vi "Main.vi"() -> ()   [LabVIEW 2026]
uses:
  Controls/Hall_Calls.ctl
  Controls/Car_Calls.ctl
  Controls/Elevator_Fleet.ctl
  Controls/Elevator_Status.ctl
  Controls/Door_Status_Enum.ctl
  Controls/Occupy_Status.ctl
  Controls/Floor_Status.ctl
  Controls/Motion_Status_Enum.ctl
  Controls/Car_Calls_Status.ctl
  Controls/Hall_Calls_Status.ctl
  Support VIs/Message Queue/Enqueue Message (Single).vi
  <vilib>/Utility/error.llb/Error Cluster From Error Code.vi
  <vilib>/ErrorRing/Error Ring.xnode
  Support VIs/Message Queue/Message Queue.lvlib
  Support VIs/User Event - Stop/User Event - Stop.lvlib
panel:
  out "Elevator Fleet":T1
  out "data":string
  in  "Exit":bool
  in  "Car Calls":T9
  in  "Hall Calls Up/Down":T10
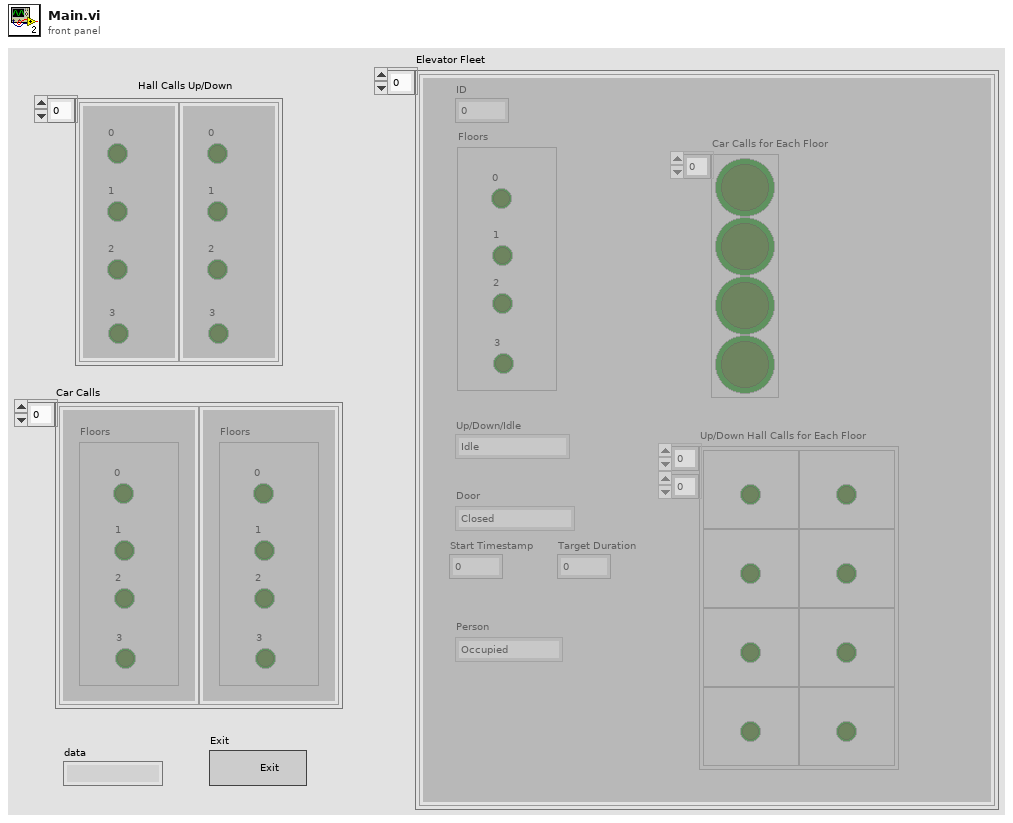
[diagram p1: front panel]
types:
  T1 = typedef "Elevator_Fleet.ctl" = T2[]
  T2 = typedef "Elevator_Status.ctl" = cluster{"Door":T3, "Person":T4, "Floors":T5, "Up/Down/Idle":T6, "Car Calls for Each Floor":T7, "Up/Down Hall Calls for Each Floor":T8, "ID":i32, "Start Timestamp":u32, "Target Duration":dbl}
  T3 = typedef "Door_Status_Enum.ctl" = enum16{"Closed", "Open", "Opening", "Closing"}
  T4 = typedef "Occupy_Status.ctl" = enum16{"Occupied", "Empty"}
  T5 = typedef "Floor_Status.ctl" = cluster{"0":bool, "1":bool, "2":bool, "3":bool}
  T6 = typedef "Motion_Status_Enum.ctl" = enum16{"Idle", "Up", "Down"}
  T7 = typedef "Car_Calls_Status.ctl" = bool[]
  T8 = typedef "Hall_Calls_Status.ctl" = cluster{bool}[][]
  T9 = typedef "Car_Calls.ctl" = cluster{"Floors":cluster{"0":bool, "1":bool, "2":bool, "3":bool}}[]
  T10 = typedef "Hall_Calls.ctl" = cluster{"0":bool, "1":bool, "2":bool, "3":bool}[]
  T11 = typedef "Message Queue.lvlib/All Message Queues.ctl" = cluster{"UI":refnum<queue>, "Acquisition":refnum<queue>, "Logging":refnum<queue>}
  T12 = enum16{"Check for Any Floor - Car Call", "Check for Specific Floor - Car Call", "Check for Any Floor - Hall Call", "Check for Specific Floor - Hall Call"}
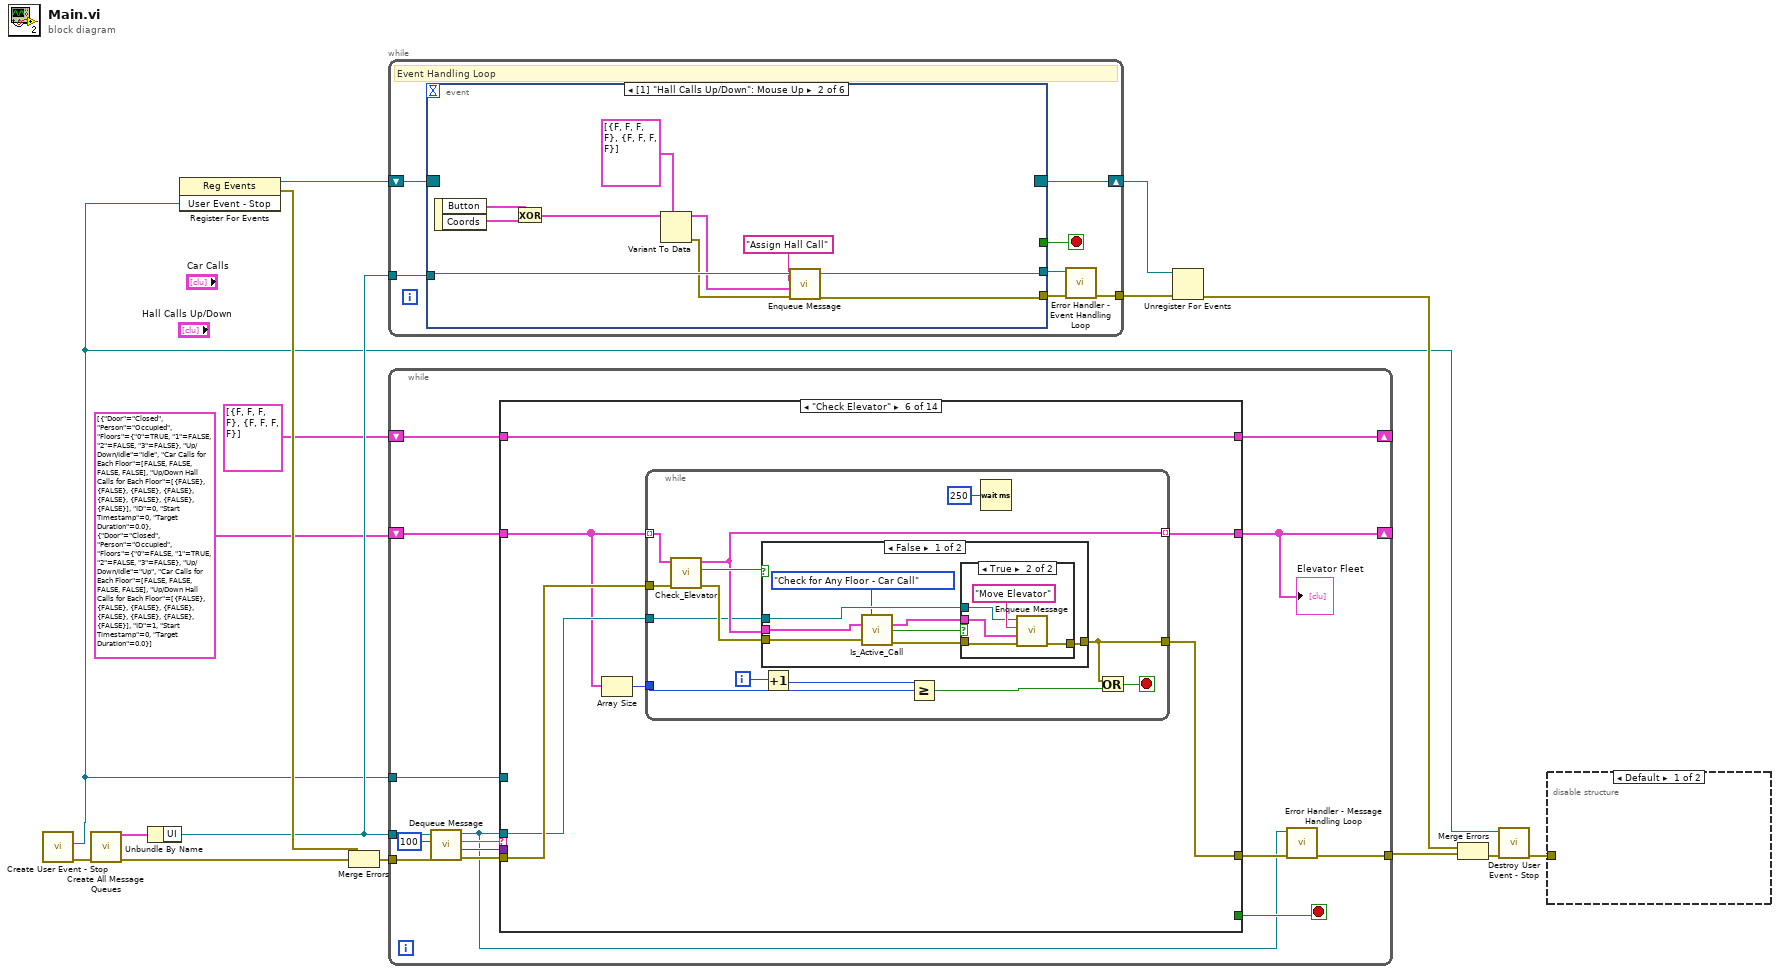
[diagram p0: block diagram]
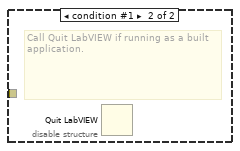
[diagram p2: hidden frame]
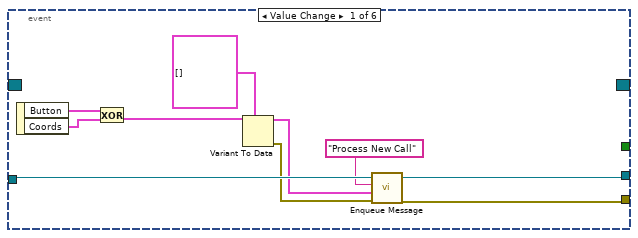
[diagram p3: hidden frame]
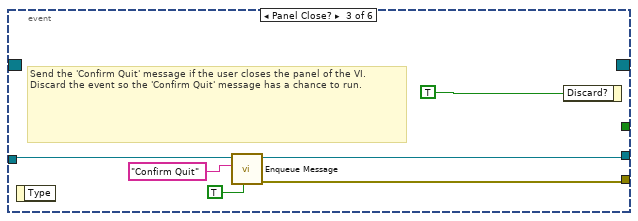
[diagram p4: hidden frame]
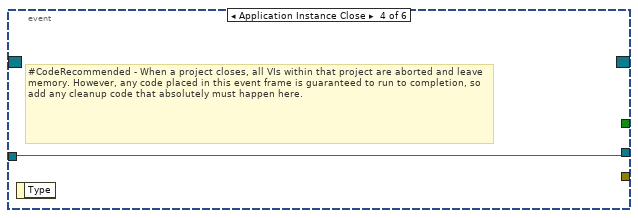
[diagram p5: hidden frame]
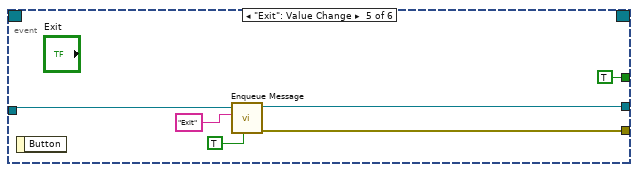
[diagram p6: hidden frame]
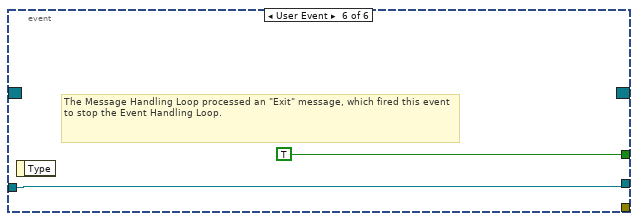
[diagram p7: hidden frame]
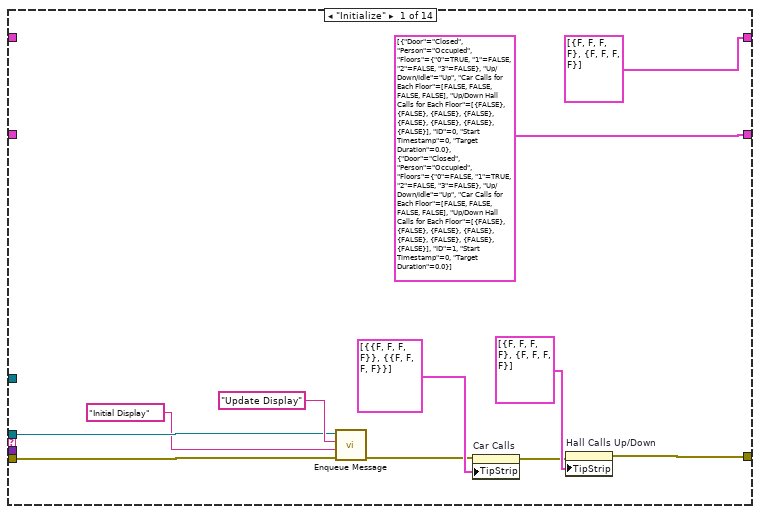
[diagram p8: hidden frame]
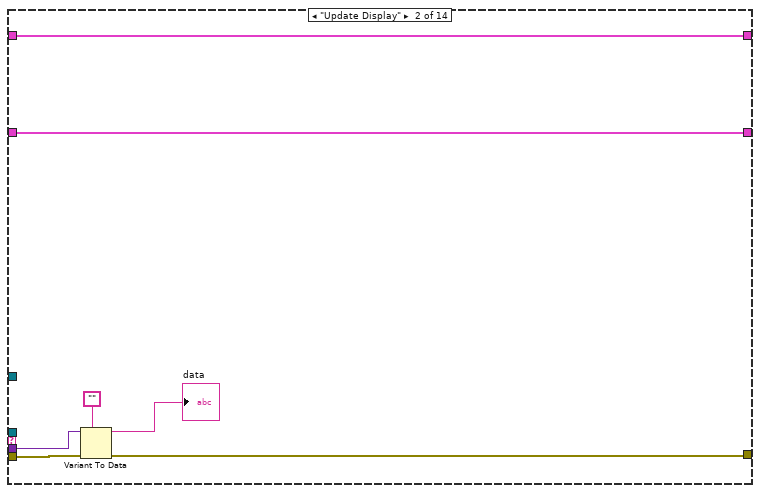
[diagram p9: hidden frame]
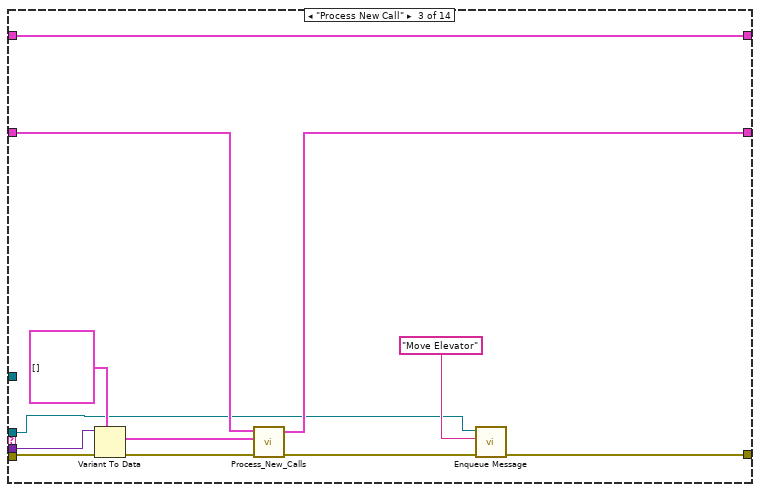
[diagram p10: hidden frame]
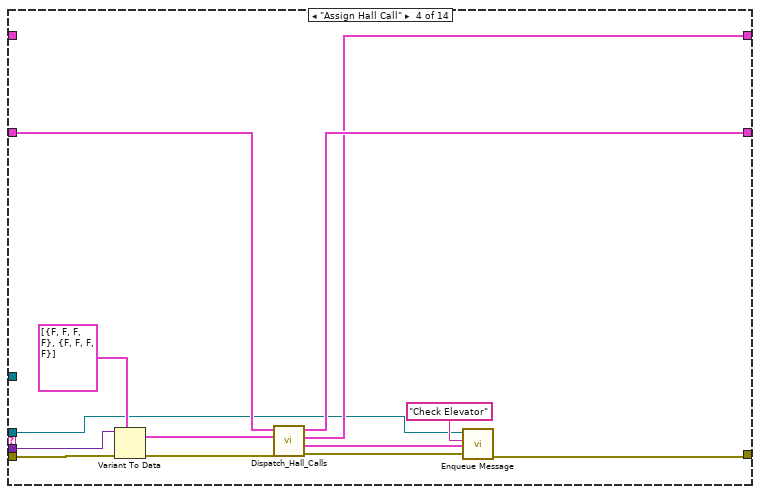
[diagram p11: hidden frame]
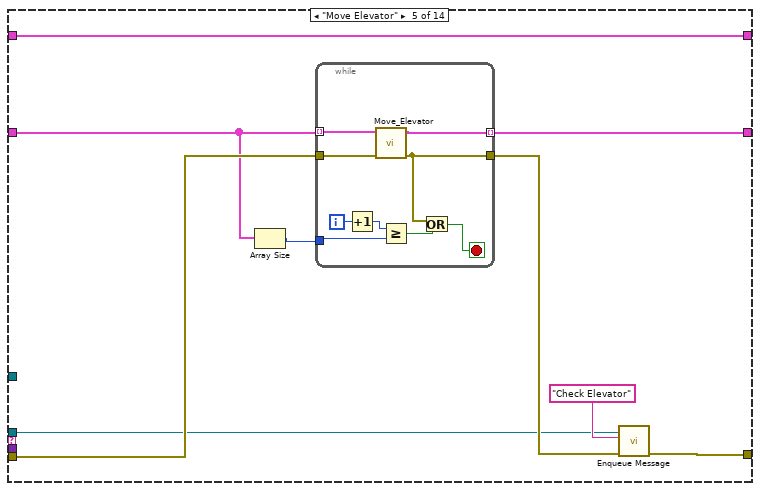
[diagram p12: hidden frame]
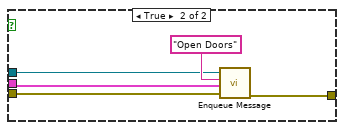
[diagram p14: hidden frame]
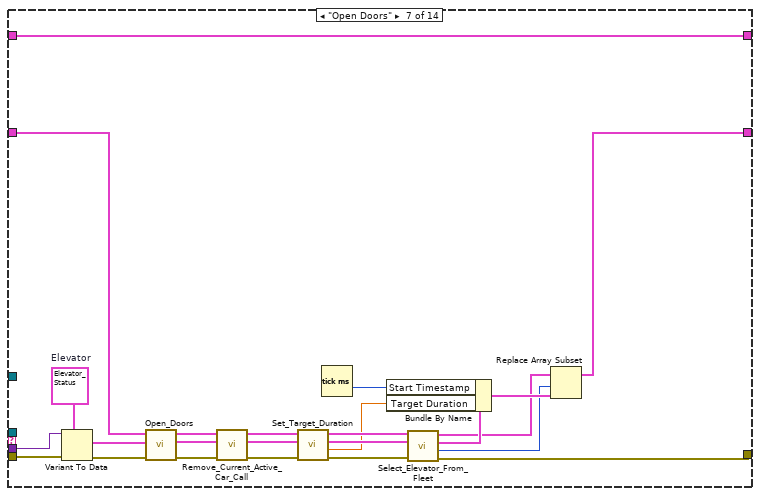
[diagram p15: hidden frame]
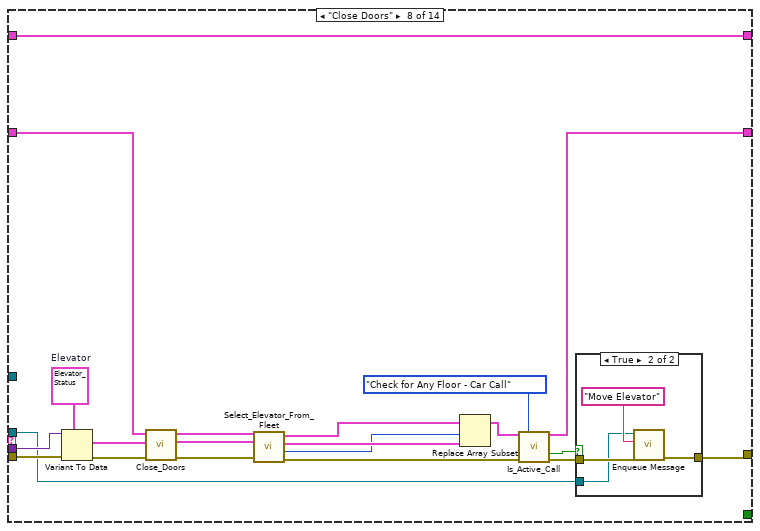
[diagram p16: hidden frame]
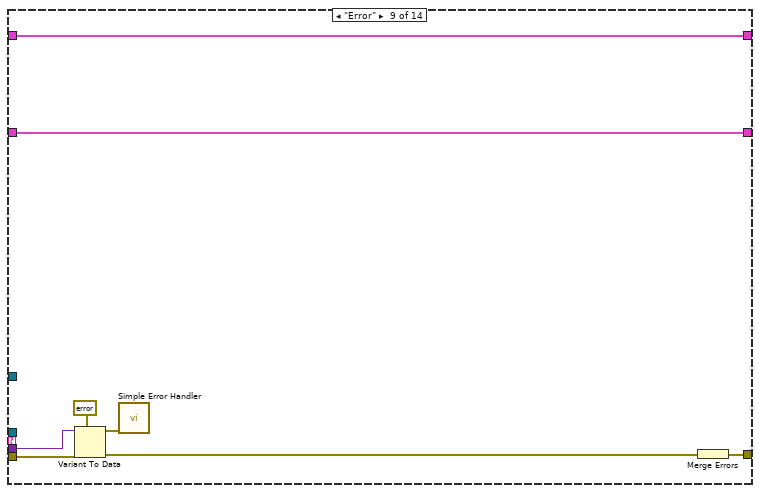
[diagram p18: hidden frame]
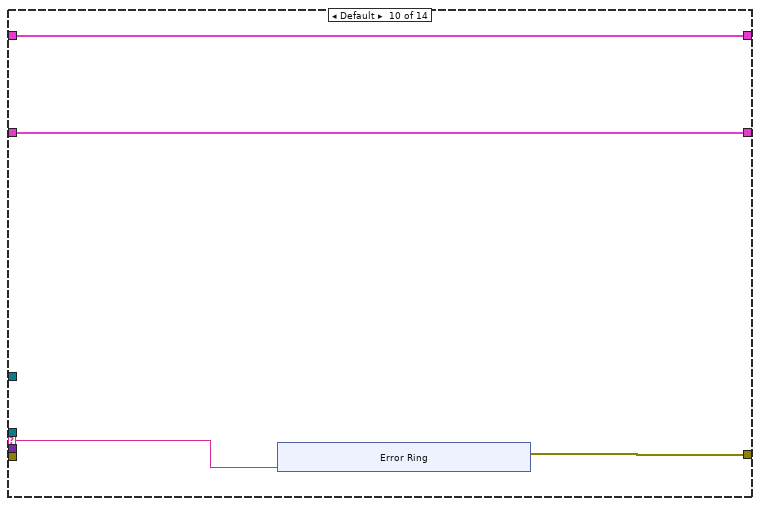
[diagram p19: hidden frame]
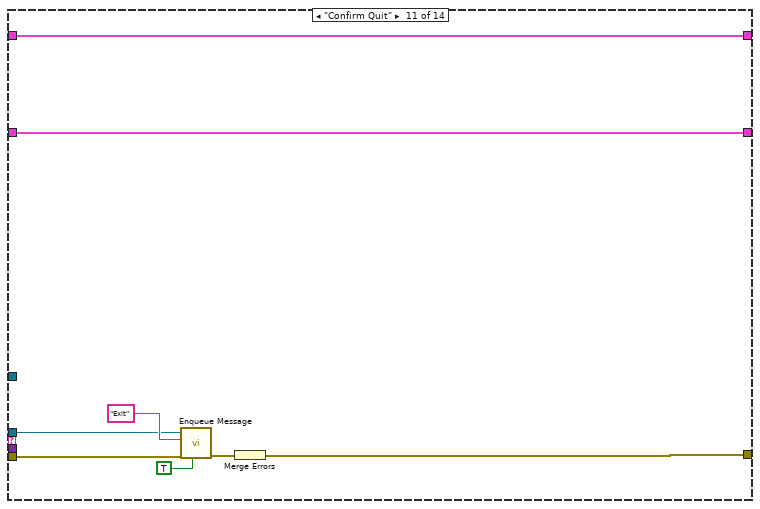
[diagram p20: hidden frame]
diagram:
  n1 = call "Create User Event - Stop.vi"() -> ("error out"=w16:errorcluster, "User Event - Stop"=w3:refnum<user-event>)  [unwired: 9 in, 1 out]
  n2 = call "Create All Message Queues.vi"("error in (no error)"=w16) -> ("error out"=w14:errorcluster, "Message Queues out"=w15:T11)  [unwired: 9 in]
  n3 = Unbundle By Name(w15) -> ("UI"=w10:refnum<queue>)
  n4 = register-events(w3) -> (reference out=w13:refnum<event-registration>, error out=w12:errorcluster)  [unwired: 2 in]
  n5 = Merge Errors(w12, w14) -> (w11:errorcluster)
  n6 = while {
    shift-right: [w23] -> w6
    shift-left: w13 -> [w18]
    tunnel: [w19] -> w7
    tunnel: w10 -> [w17]
    stop <- w21 stop-if-true
    # "Event Handling Loop"
    n7 = event shown="[1] \"Hall Calls Up/Down\": Mouse Up" {
      selector: w18 -> [_ _ _ _ _ _]
      dyn-events: [_ _ _ _ _ _] -> w23
      timeout: _ -> [_ _ _ _ _ _]
      tunnel: [_ _ _ _ TRUE ("Discard?") TRUE ("Discard?")] -> w21
      tunnel: [w32 w42 w48 _ w56 _] -> w22
      tunnel: [w33 w43 w47 w50 w55 w57] -> w20
      tunnel: w17 -> [w31 w41 w44 w50 w52 w57]
      event Value Change {
        n8 = event-data() -> ("Button"=w26:T9, "Coords"=w25:T9)  [unwired: 1 in]
        n9 = Exclusive Or(1:w25, 2:w26) -> (0:w24:T9)
        n10 = Variant To Data(type=T9 [] ("x .xor. y?"), Variant=w24) -> (data=w29:T9, error out=w28:errorcluster)  [unwired: 1 in]
        n11 = call-poly "Enqueue Message.vi"("error in (no error)"=w28, "Message Data"=w29, "Message"="Process New Call", "Message Queue"=w31) -> ("error out"=w32:errorcluster, "dup Message Queue"=w33:refnum<queue>)  [unwired: 6 in]
      }
      event Value Change {
        n12 = event-data() -> ("Button"=w37:T10, "Coords"=w36:T10)  [unwired: 1 in]
        n13 = Exclusive Or(1:w36, 2:w37) -> (0:w35:T10)
        n14 = Variant To Data(type=T10 [{"0"=FALSE, "1"=FALSE, "2"=FALSE, "3"=FALSE}, {"0"=FALSE, "1"=FALSE, "2"=FALSE, "3"=FALSE}] ("x .xor. y?"), Variant=w35) -> (data=w39:T10, error out=w38:errorcluster)  [unwired: 1 in]
        n15 = call-poly "Enqueue Message.vi"("error in (no error)"=w38, "Message Data"=w39, "Message"="Assign Hall Call", "Message Queue"=w41) -> ("error out"=w42:errorcluster, "dup Message Queue"=w43:refnum<queue>)  [unwired: 6 in]
      }
      event Panel Close? {
        # "Send the 'Confirm Quit' message if the user closes the panel of the VI. Discard the event so the 'Confirm Quit' message has a chance to run."
        n16 = event-data() -> ()  [unwired: 1 in, 1 out]
        n17 = call-poly "Enqueue Message.vi"("Priority Message? (F)"=TRUE, "Message"="Confirm Quit", "Message Queue"=w44) -> ("error out"=w48:errorcluster, "dup Message Queue"=w47:refnum<queue>)  [unwired: 7 in]
        n18 = event-data("Discard?"=TRUE) -> ()  [unwired: 1 in, 1 out]
      }
      event Application Instance Close {
        # "#CodeRecommended - When a project closes, all VIs within that project are aborted and leave memory. However, any code placed in this event frame is guaranteed to run to completion, so add any cleanup code that absolutely must happen here."
        n19 = event-data() -> ()  [unwired: 1 in, 1 out]
      }
      event "Exit": Value Change {
        n20 = event-data() -> ()  [unwired: 1 in, 1 out]
        n21 = call-poly "Enqueue Message.vi"("Priority Message? (F)"=TRUE, "Message"="Exit", "Message Queue"=w52) -> ("error out"=w56:errorcluster, "dup Message Queue"=w55:refnum<queue>)  [unwired: 7 in]
      }
      event User Event {
        # "The Message Handling Loop processed an \"Exit\" message, which fired this event to stop the Event Handling Loop."
        n22 = event-data() -> ()  [unwired: 1 in, 1 out]
      }
    }
    n23 = call "Error Handler - Event Handling Loop.vi"("error in (no error)"=w22, "Message Queue"=w20) -> ("dup error in"=w19:errorcluster)  [unwired: 8 in, 1 out]
  }
  n24 = while {
    tunnel: w10 -> [w72]
    tunnel: w11 -> [w71]
    tunnel: w3 -> [w67]
    tunnel: [w65] -> w8
    shift-right: [w63] -> _
    shift-left: T1 [{"Door"=enum."Closed", "Person"=enum."Occupied", "Floors"={"0"=TRUE, "1"=FALSE, "2"=FALSE, "3"=FALSE}, "Up/Down/Idle"=enum."Idle", "Car Calls for Each Floor"=[FALSE, FALSE, FALSE, FALSE], "Up/Down Hall Calls for Each Floor"=[[{FALSE}, {FALSE}], [{FALSE}, {FALSE}], [{FALSE}, {FALSE}], [{FALSE}, {FALSE}]], "ID"=0, "Start Timestamp"=0, "Target Duration"=0.0}, {"Door"=enum."Closed", "Person"=enum."Occupied", "Floors"={"0"=FALSE, "1"=TRUE, "2"=FALSE, "3"=FALSE}, "Up/Down/Idle"=enum."Up", "Car Calls for Each Floor"=[FALSE, FALSE, FALSE, FALSE], "Up/Down Hall Calls for Each Floor"=[[{FALSE}, {FALSE}], [{FALSE}, {FALSE}], [{FALSE}, {FALSE}], [{FALSE}, {FALSE}]], "ID"=1, "Start Timestamp"=0, "Target Duration"=0.0}] ("Elevator Fleet") -> [w73]
    shift-right: [w61] -> _
    shift-left: T10 [{"0"=FALSE, "1"=FALSE, "2"=FALSE, "3"=FALSE}, {"0"=FALSE, "1"=FALSE, "2"=FALSE, "3"=FALSE}] ("x .xor. y?") -> [w62]
    stop <- w64 stop-if-true
    n25 = call "Dequeue Message.vi"("error in (no error)"=w71, "Timeout (ms)"=100, "Message Queue"=w72) -> ("error out"=w69:errorcluster, "Message Data"=w68:variant, "Message"=w70:string, "dup Message Queue"=w60:refnum<queue>)  [unwired: 5 in]
    n26 = case shown="\"Check Elevator\"" w70 {
      selector: w70 -> [_ _ _ _ _ _ _ _ _ w235 _ _ _ _]
      tunnel: w73 -> [_ w86 w98 w113 w118 w136 w193 w214 w225 w233 w244 w252 w257 w300]
      tunnel: w60 -> [w82 _ w92 w105 w119 w137 _ w199 _ _ w245 _ w260 w302]
      tunnel: w69 -> [w83 w90 w100 w116 w121 w140 w196 w217 w229 _ w246 w254 w259 w298]
      tunnel: w68 -> [_ w89 w102 w115 _ _ w195 w216 w228 _ _ _ _ w301]
      tunnel: [w74 w88 w95 w108 w122 w138 w185 w201 w226 w234 w247 w253 w258 w305] -> w66
      tunnel: w67 -> [_ _ _ _ _ _ _ _ _ _ _ _ _ w303]
      tunnel: [_ _ _ _ _ _ _ _ _ _ _ _ _ TRUE] -> w64
      tunnel: [T1 [{"Door"=enum."Closed", "Person"=enum."Occupied", "Floors"={"0"=TRUE, "1"=FALSE, "2"=FALSE, "3"=FALSE}, "Up/Down/Idle"=enum."Up", "Car Calls for Each Floor"=[FALSE, FALSE, FALSE, FALSE], "Up/Down Hall Calls for Each Floor"=[[{FALSE}, {FALSE}], [{FALSE}, {FALSE}], [{FALSE}, {FALSE}], [{FALSE}, {FALSE}]], "ID"=0, "Start Timestamp"=0, "Target Duration"=0.0}, {"Door"=enum."Closed", "Person"=enum."Occupied", "Floors"={"0"=FALSE, "1"=TRUE, "2"=FALSE, "3"=FALSE}, "Up/Down/Idle"=enum."Up", "Car Calls for Each Floor"=[FALSE, FALSE, FALSE, FALSE], "Up/Down Hall Calls for Each Floor"=[[{FALSE}, {FALSE}], [{FALSE}, {FALSE}], [{FALSE}, {FALSE}], [{FALSE}, {FALSE}]], "ID"=1, "Start Timestamp"=0, "Target Duration"=0.0}] ("Elevator Fleet") w86 w97 w114 w124 w139 w187 w200 w225 w233 w244 w252 w255 w300] -> w63
      tunnel: w62 -> [_ w85 w103 _ w125 w141 w197 w218 w224 w232 w243 w251 w261 w299]
      tunnel: [T10 [{"0"=FALSE, "1"=FALSE, "2"=FALSE, "3"=FALSE}, {"0"=FALSE, "1"=FALSE, "2"=FALSE, "3"=FALSE}] ("x .xor. y?") w85 w103 w110 w125 w141 w197 w218 w224 w232 w243 w251 w261 w299] -> w61
      frame "Initialize" {
        n27 = call-poly "Enqueue Message.vi"("error in (no error)"=w83, "Message Data"="Initial Display" ("Message"), "Message"="Update Display", "Message Queue"=w82) -> ("error out"=w77:errorcluster)  [unwired: 6 in, 1 out]
        n28 = property on="Car Calls" class="Arr (strict)"(error in=w77, "TipStrip"=T9 [{"Floors"={"0"=FALSE, "1"=FALSE, "2"=FALSE, "3"=FALSE}}, {"Floors"={"0"=FALSE, "1"=FALSE, "2"=FALSE, "3"=FALSE}}] ("Car Calls")) -> (error out=w75:errorcluster)  [unwired: 1 in, 1 out]
        n29 = property on="Hall Calls Up/Down" class="Arr (strict)"(error in=w75, "TipStrip"=T10 [{"0"=FALSE, "1"=FALSE, "2"=FALSE, "3"=FALSE}, {"0"=FALSE, "1"=FALSE, "2"=FALSE, "3"=FALSE}] ("Hall Calls Up/Down")) -> (error out=w74:errorcluster)  [unwired: 1 in, 1 out]
      }
      frame "Update Display" {
        n30 = Variant To Data(error in=w90, type="", Variant=w89) -> (data=→"data":string, error out=w88:errorcluster)
      }
      frame "Process New Call" {
        n31 = Variant To Data(error in=w100, type=T9 [] ("x .xor. y?"), Variant=w102) -> (data=w99:T9, error out=w94:errorcluster)
        n32 = call "Process_New_Calls.vi"("error in (no error)"=w94, "Car Calls in"=w99, "Elevator Fleet in"=w98) -> ("error out"=w93:errorcluster, "Elevator Fleet out"=w97:T1)  [unwired: 7 in]
        n33 = call-poly "Enqueue Message.vi"("error in (no error)"=w93, "Message"="Move Elevator", "Message Queue"=w92) -> ("error out"=w95:errorcluster)  [unwired: 7 in, 1 out]
      }
      frame "Assign Hall Call" {
        n34 = Variant To Data(error in=w116, type=T10 [{"0"=FALSE, "1"=FALSE, "2"=FALSE, "3"=FALSE}, {"0"=FALSE, "1"=FALSE, "2"=FALSE, "3"=FALSE}] ("x .xor. y?"), Variant=w115) -> (data=w111:T10, error out=w107:errorcluster)
        n35 = call "Dispatch_Hall_Calls.vi"("error in (no error)"=w107, "Hall Calls Up/Down In"=w111, "Elevator Fleet in"=w113) -> ("error out"=w106:errorcluster, "Elevator Called"=w104:T2, "Hall Calls Up/Down Out"=w110:T10, "Elevator Fleet out"=w114:T1)  [unwired: 5 in]
        n36 = call-poly "Enqueue Message.vi"("error in (no error)"=w106, "Message Data"=w104, "Message"="Check Elevator", "Message Queue"=w105) -> ("error out"=w108:errorcluster)  [unwired: 6 in, 1 out]
      }
      frame "Move Elevator" {
        n37 = Array Size(array=w118) -> (size(s)=w117:i32)
        n38 = while {
          tunnel: w118 -> [w134] mode=indexing
          tunnel: [w133] -> w124 mode=indexing
          tunnel: w121 -> [w132]
          tunnel: [w129] -> w120
          tunnel: w117 -> [w131]
          i -> [w127]
          stop <- w130 stop-if-true
          n39 = Increment(x=w127) -> (x+1=w126:i32)
          n40 = call "Move_Elevator.vi"("error in (no error)"=w132, "Elevator in"=w134) -> ("error out"=w129:errorcluster, "Elevator out"=w133:T2)  [unwired: 8 in]
          n41 = Greater Or Equal?(x=w126, y=w131) -> (x >= y?=w128:bool)
          n42 = Or(x=w129, y=w128) -> (x .or. y?=w130:bool)
        }
        n43 = call-poly "Enqueue Message.vi"("error in (no error)"=w120, "Message"="Check Elevator", "Message Queue"=w119) -> ("error out"=w122:errorcluster)  [unwired: 7 in, 1 out]
      }
      frame "Check Elevator" {
        n44 = Array Size(array=w136) -> (size(s)=w135:i32)
        n45 = while {
          tunnel: w140 -> [w154]
          tunnel: [w151] -> w139 mode=indexing
          tunnel: [w147] -> w138
          tunnel: w137 -> [w150]
          tunnel: w136 -> [w149] mode=indexing
          tunnel: w135 -> [w148]
          i -> [w143]
          stop <- w145 stop-if-true
          n46 = call "Check_Elevator.vi"("error in (no error)"=w154, "Elevator in"=w149) -> ("error out"=w152:errorcluster, "Open Doors?"=w153:bool, "Elevator out"=w151:T2)  [unwired: 7 in]
          n47 = case shown="False" w153 {
            tunnel: w152 -> [w161 w172]
            tunnel: [w157 w171] -> w147
            tunnel: w151 -> [w159 w170]
            tunnel: w150 -> [w162 w169]
            frame False {
              n48 = call "Is_Active_Call.vi"("Enum"=T12."Check for Any Floor - Car Call", "Elevator in"=w159, "error in (no error)"=w161) -> ("Elevator out"=w156:T2, "Active Call?"=w158:bool, "error out"=w160:errorcluster)  [unwired: 8 in, 2 out]
              n49 = case shown="True" w158 {
                tunnel: w162 -> [_ w167]
                tunnel: w160 -> [w163 w166]
                tunnel: [w163 w165] -> w157
                tunnel: w156 -> [_ w164]
                frame False {
                }
                frame True {
                  n50 = call-poly "Enqueue Message.vi"("error in (no error)"=w166, "Message Data"=w164, "Message"="Move Elevator", "Message Queue"=w167) -> ("error out"=w165:errorcluster)  [unwired: 6 in, 1 out]
                }
              }
            }
            frame True {
              n51 = call-poly "Enqueue Message.vi"("error in (no error)"=w172, "Message Data"=w170, "Message"="Open Doors", "Message Queue"=w169) -> ("error out"=w171:errorcluster)  [unwired: 6 in, 1 out]
            }
          }
          n52 = Increment(x=w143) -> (x+1=w142:i32)
          n53 = Greater Or Equal?(x=w142, y=w148) -> (x >= y?=w146:bool)
          n54 = Wait (ms)(milliseconds to wait=u32 250) -> ()  [unwired: 1 out]
          n55 = Or(x=w147, y=w146) -> (x .or. y?=w145:bool)
        }
      }
      frame "Open Doors" {
        w194 = T2 {"Door"=enum."Closed", "Person"=enum."Occupied", "Floors"={"0"=FALSE, "1"=FALSE, "2"=FALSE, "3"=FALSE}, "Up/Down/Idle"=enum."Idle", "Car Calls for Each Floor"=[], "Up/Down Hall Calls for Each Floor"=[], "ID"=0, "Start Timestamp"=0, "Target Duration"=0.0}  # Elevator
        n56 = Variant To Data(error in=w196, type=w194, Variant=w195) -> (data=w192:T2, error out=w191:errorcluster)
        n57 = call "Open_Doors.vi"("error in (no error)"=w191, "Elevator in"=w192, "Elevator Fleet in"=w193) -> ("error out"=w175:errorcluster, "Elevator out"=w177:T2, "Elevator Fleet out"=w179:T1)  [unwired: 6 in]
        n58 = call "Remove_Current_Active_Car_Call.vi"("error in (no error)"=w175, "Elevator in"=w177, "Elevator Fleet in"=w179) -> ("error out"=w174:errorcluster, "Elevator out"=w176:T2, "Elevator Fleet out"=w178:T1)  [unwired: 6 in]
        n59 = call "Set_Target_Duration.vi"("error in (no error)"=w174, "Elevator in"=w176, "Elevator Fleet in"=w178) -> ("error out"=w186:errorcluster, "Target Duration"=w181:dbl, "Elevator out"=w182:T2, "Elevator Fleet out"=w183:T1)  [unwired: 5 in]
        n60 = Tick Count (ms)() -> (millisecond timer value=w189:u32)
        n61 = call "Select_Elevator_From_Fleet.vi"("error in (no error)"=w186, "Elevator in"=w182, "Elevator Fleet in"=w183) -> ("error out"=w185:errorcluster, "ID"=w184:i32, "Elevator out"=w190:T2, "Elevator Fleet out"=w180:T1)  [unwired: 5 in]
        n62 = Bundle By Name(cluster=w190, "Start Timestamp"=w189, "Target Duration"=w181) -> (w188:T2)
        n63 = Replace Array Subset(array=w180, new element=w188, index=w184) -> (w187:T1)
      }
      frame "Close Doors" {
        w215 = T2 {"Door"=enum."Closed", "Person"=enum."Occupied", "Floors"={"0"=FALSE, "1"=FALSE, "2"=FALSE, "3"=FALSE}, "Up/Down/Idle"=enum."Idle", "Car Calls for Each Floor"=[], "Up/Down Hall Calls for Each Floor"=[], "ID"=0, "Start Timestamp"=0, "Target Duration"=0.0}  # Elevator
        n64 = Variant To Data(error in=w217, type=w215, Variant=w216) -> (data=w213:T2, error out=w212:errorcluster)
        n65 = call "Close_Doors.vi"("error in (no error)"=w212, "Elevator in"=w213, "Elevator Fleet in"=w214) -> ("error out"=w209:errorcluster, "Elevator out"=w210:T2, "Elevator Fleet out"=w211:T1)  [unwired: 6 in]
        n66 = call "Select_Elevator_From_Fleet.vi"("error in (no error)"=w209, "Elevator in"=w210, "Elevator Fleet in"=w211) -> ("error out"=w205:errorcluster, "ID"=w206:i32, "Elevator out"=w207:T2, "Elevator Fleet out"=w208:T1)  [unwired: 5 in]
        n67 = Replace Array Subset(array=w208, new element=w207, index=w206) -> (w204:T1)
        n68 = call "Is_Active_Call.vi"("Elevator Fleet in"=w204, "Enum"=T12."Check for Any Floor - Car Call", "error in (no error)"=w205) -> ("Elevator Fleet out"=w200:T1, "Active Call?"=w203:bool, "error out"=w202:errorcluster)  [unwired: 8 in, 2 out]
        n69 = case shown="True" w203 {
          tunnel: w202 -> [w219 w222]
          tunnel: [w219 w221] -> w201
          tunnel: w199 -> [_ w220]
          frame False {
          }
          frame True {
            n70 = call-poly "Enqueue Message.vi"("error in (no error)"=w222, "Message"="Move Elevator", "Message Queue"=w220) -> ("error out"=w221:errorcluster)  [unwired: 7 in, 1 out]
          }
        }
      }
      frame "Error" {
        n71 = Variant To Data(error in=w229, type=errorcluster {"status"=FALSE, "code"=0, "source"=""} ("error constant"), Variant=w228) -> (data=w231:errorcluster, error out=w227:errorcluster)
        n72 = call <vilib>:"Simple Error Handler.vi"("error in (no error)"=w231) -> ()  [unwired: 4 in, 5 out]
        n73 = Merge Errors(w227) -> (w226:errorcluster)
      }
      frame Default {
        n74 = xnode "Error Ring"("parameter 0"=w235) -> ("error out"=w234:errorcluster)
      }
      frame "Confirm Quit" {
        n75 = call-poly "Enqueue Message.vi"("Priority Message? (F)"=TRUE, "error in (no error)"=w246, "Message"="Exit", "Message Queue"=w245) -> ("error out"=w248:errorcluster)  [unwired: 6 in, 1 out]
        n76 = Merge Errors(w248) -> (w247:errorcluster)
      }
      frame "---Copy This Frame---" {
        n77 = Merge Errors(w254) -> (w253:errorcluster)
      }
      frame "Timeout" {
        n78 = Array Size(array=w257) -> (size(s)=w256:i32)
        n79 = while {
          tunnel: w257 -> [w263] mode=indexing
          tunnel: w260 -> [w273]
          tunnel: w259 -> [w272]
          tunnel: [w269] -> w258
          tunnel: w256 -> [w271]
          tunnel: [w262] -> w255 mode=indexing
          i -> [w265]
          stop <- w270 stop-if-true
          n80 = Unbundle By Name(w263) -> ("Start Timestamp"=w266:u32, "Target Duration"=w274:dbl)
          n81 = Increment(x=w265) -> (x+1=w264:i32)
          n82 = Greater Or Equal?(x=w264, y=w271) -> (x >= y?=w268:bool)
          n83 = Not Equal To 0?(x=w266) -> (x != 0?=w267:bool)
          n84 = case shown="True" w267 {
            tunnel: w274 -> [_ w286]
            tunnel: w273 -> [_ w282]
            tunnel: w272 -> [w276 w281]
            tunnel: [w276 w280] -> w269
            tunnel: w266 -> [_ w279]
            tunnel: w263 -> [w275 w278]
            tunnel: [w275 w277] -> w262
            frame False {
            }
            frame True {
              n85 = Tick Count (ms)() -> (millisecond timer value=w287:u32)
              n86 = Subtract(x=w287, y=w279) -> (x-y=w284:u32)
              n87 = To Double Precision Float(number=w284) -> (double precision float=w285:dbl)
              n88 = Greater Or Equal?(x=w285, y=w286) -> (x >= y?=w283:bool)
              n89 = case shown="True" w283 {
                tunnel: w281 -> [w289 w295]
                tunnel: [w289 w294] -> w280
                tunnel: w282 -> [_ w293]
                tunnel: w278 -> [w288 w292]
                tunnel: [w288 w290] -> w277
                frame False {
                }
                frame True {
                  n90 = Bundle By Name(cluster=w292, "Start Timestamp"=u32 0) -> (w290:T2)
                  n91 = call-poly "Enqueue Message.vi"("error in (no error)"=w295, "Message Data"=w290, "Message"="Close Doors", "Message Queue"=w293) -> ("error out"=w294:errorcluster)  [unwired: 6 in, 1 out]
                }
              }
            }
          }
          n92 = Or(x=w269, y=w268) -> (x .or. y?=w270:bool)
        }
      }
      frame "Exit" {
        # "Stop the VI"
        # "Release the message queue reference"
        n93 = Variant To Data(error in=w298, type=errorcluster {"status"=FALSE, "code"=0, "source"=""} ("error constant"), Variant=w301) -> (data=w306:errorcluster, error out=w297:errorcluster)
        n94 = call <vilib>:"Simple Error Handler.vi"("error in (no error)"=w306) -> ()  [unwired: 4 in, 5 out]
        n95 = call "Fire User Event - Stop.vi"("User Event - Stop"=w303) -> ("error out"=w308:errorcluster)  [unwired: 10 in]
        n96 = Release Queue(queue=w302, error in (no error)=w297) -> (error out=w309:errorcluster)  [unwired: 1 in, 2 out]
        n97 = Merge Errors(w308, w309) -> (w305:errorcluster)
      }
    }
    "Elevator Fleet" <- w63
    n98 = call "Error Handler - Message Handling Loop.vi"("error in (no error)"=w66, "Message Queue"=w60) -> ("dup error in"=w65:errorcluster)  [unwired: 8 in, 1 out]
  }
  n99 = Unregister For Events(event registration refnum=w6, error in=w7) -> (error out=w5:errorcluster)
  n100 = Merge Errors(w5, w8) -> (w9:errorcluster)
  n101 = call "Destroy User Event - Stop.vi"("error in (no error)"=w9, "User Event - Stop"=w3) -> ("error out"=w4:errorcluster)  [unwired: 9 in]
  n102 = disable-structure shown="Default" {
    disable-tunnel: w4 -> [_ _]
    frame condition #0 (active) {
    }
    frame condition #1 {
      # "Call Quit LabVIEW if running as a built application."
      n103 = Quit LabVIEW() -> ()  [unwired: 1 in]
    }
  }
